vi "INI_Read LV INI Settings.vi"(8 "error in":errorcluster) -> (0 "error out":errorcluster, 3 "LabVIEW INI Settings":cluster{"Scripting":bool, "Private":bool})   [LabVIEW 2023]
doc: "Read LV ini file and determine is Scripting and Private settings are active.\n\nThis VI asumes that labview.ini is in the application directory. It may not be. By default it is on Windows. The function LV provides to determine the ini file path is password protected and can't be backsaved for use in prior versions. If this turns out to fail for multiple users, we can work on correcting this."
uses:
  <vilib>/Utility/config.llb/Read Key (Boolean).vi
  <vilib>/Utility/config.llb/NI_LVConfig.lvlib
  <userlib>/_OpenG.lib/file/file.llb/openg_file.lvlib
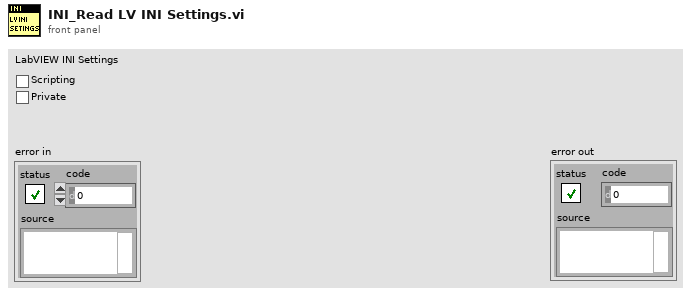
[diagram p1: front panel]
types:
  T1 = typedef "NI_LVConfig.lvlib/Config Data RefNum.ctl" = refnum<k1>
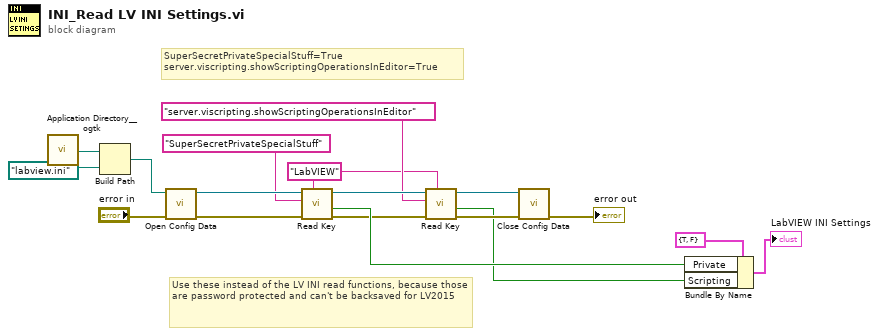
[diagram p0: block diagram]
diagram:
  w5 = "LabVIEW" ("section")
  # "Use these instead of the LV INI read functions, because those are password protected and can't be backsaved for LV2015"
  # "SuperSecretPrivateSpecialStuff=True\nserver.viscripting.showScriptingOperationsInEditor=True"
  n1 = call <userlib>:"Application Directory__ogtk.vi"() -> ("Application Directory (+ Relative)"=w3:path)  [unwired: 1 in]
  n2 = Build Path(base path=w3, name or relative path=path "labview.ini") -> (appended path=w1:path)
  n3 = call <vilib>:"Open Config Data.vi"("error in (no error)"="error in", "configuration file path"=w1) -> ("error out"=w16:errorcluster, "refnum"=w15:T1)  [unwired: 7 in, 1 out]
  n4 = call-poly <vilib>:"Read Key.vi"("section"=w5, "error in (no error)"=w16, "key"="SuperSecretPrivateSpecialStuff" ("regular expression"), "refnum"=w15) -> ("error out"=w10:errorcluster, "value"=w11:bool, "refnum out"=w9:T1)  [unwired: 4 in, 1 out]
  n5 = call-poly <vilib>:"Read Key.vi"("section"=w5, "error in (no error)"=w10, "key"="server.viscripting.showScriptingOperationsInEditor" ("regular expression"), "refnum"=w9) -> ("error out"=w8:errorcluster, "value"=w4:bool, "refnum out"=w7:T1)  [unwired: 4 in, 1 out]
  n6 = call <vilib>:"Close Config Data.vi"("error in (no error)"=w8, "refnum"=w7) -> ("error out"=→"error out":errorcluster)  [unwired: 8 in, 1 out]
  n7 = Bundle By Name(cluster=cluster{"Scripting":bool, "Private":bool} {"Scripting"=TRUE, "Private"=FALSE} ("LabVIEW INI Settings"), "Private"=w11, "Scripting"=w4) -> (→"LabVIEW INI Settings":cluster{"Scripting":bool, "Private":bool})
